vi "Principal.vi"() -> ()   [LabVIEW 2018]
panel:
  out "Turner Indicator":dbl(knob) scale=80.0..120.0 scale format="%#_50g"
  out "SHARP":bool
  out "TUNED":bool
  out "FLAT":bool
  in  "Choosing the string":i32(knob) scale=0.0..5.0
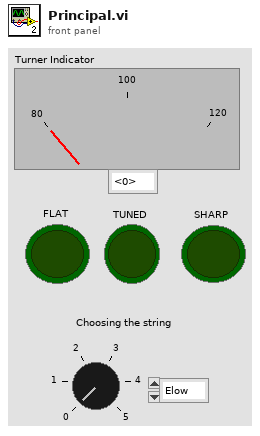
[diagram p1: front panel]
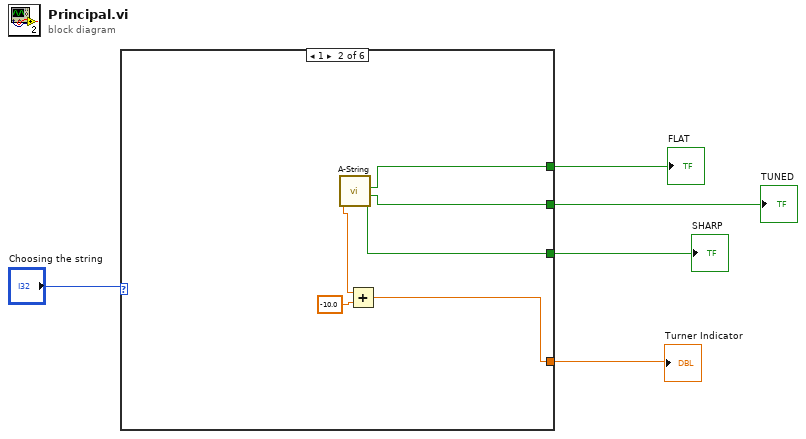
[diagram p0: block diagram]
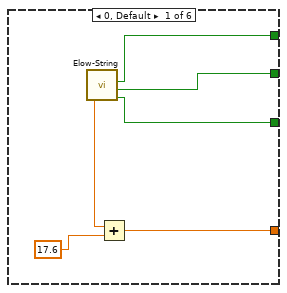
[diagram p2: hidden frame]
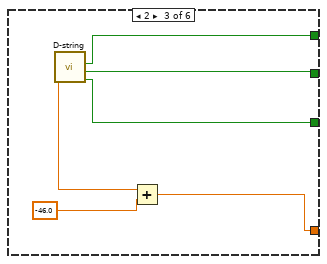
[diagram p3: hidden frame]
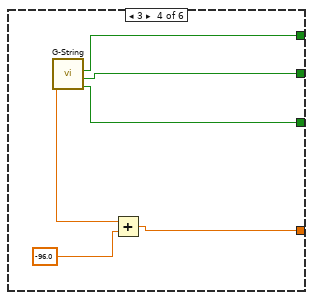
[diagram p4: hidden frame]
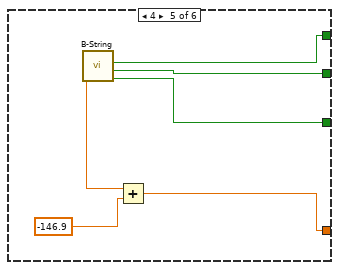
[diagram p5: hidden frame]
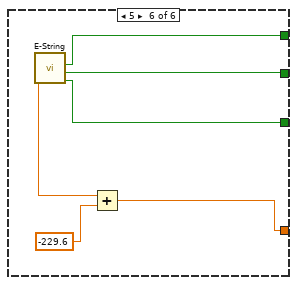
[diagram p6: hidden frame]
diagram:
  n1 = case shown="1" "Choosing the string" {
    tunnel: [w10 w16 w22 w26 w31 w38] -> w4
    tunnel: [w9 w15 w19 w29 w33 w41] -> w3
    tunnel: [w8 w14 w20 w28 w34 w40] -> w2
    tunnel: [w7 w13 w21 w27 w35 w39] -> w1
    frame 0, Default {
      n2 = call "Elow-String.vi"() -> ("SHARP"=w7:bool, "TUNED"=w8:bool, "FLAT"=w9:bool, "FREQ at maximum"=w6:dbl)  [unwired: 3 in, 1 out]
      n3 = Add(x=w6, y=17.6) -> (x+y=w10:dbl)
    }
    frame 1 {
      n4 = call "A-String.vi"() -> ("SHARP"=w13:bool, "TUNED"=w14:bool, "FLAT"=w15:bool, "FREQ at maximum"=w12:dbl)  [unwired: 6 in, 1 out]
      n5 = Add(x=w12, y=-10.0) -> (x+y=w16:dbl)
    }
    frame 2 {
      n6 = call "D-string.vi"() -> ("SHARP"=w21:bool, "TUNED"=w20:bool, "FLAT"=w19:bool, "FREQ at maximum"=w18:dbl)  [unwired: 7 in, 1 out]
      n7 = Add(x=w18, y=-46.0) -> (x+y=w22:dbl)
    }
    frame 3 {
      n8 = call "G-String.vi"() -> ("SHARP"=w27:bool, "TUNED"=w28:bool, "FLAT"=w29:bool, "FREQ at maximum"=w24:dbl)  [unwired: 5 in, 1 out]
      n9 = Add(x=w24, y=-96.0) -> (x+y=w26:dbl)
    }
    frame 4 {
      n10 = call "B-String.vi"() -> ("SHARP"=w35:bool, "TUNED"=w34:bool, "FLAT"=w33:bool, "FREQ at maximum"=w30:dbl)  [unwired: 5 in, 1 out]
      n11 = Add(x=w30, y=-146.9) -> (x+y=w31:dbl)
    }
    frame 5 {
      n12 = call "E-String.vi"() -> ("SHARP"=w39:bool, "TUNED"=w40:bool, "FLAT"=w41:bool, "FREQ at maximum"=w36:dbl)  [unwired: 6 in, 1 out]
      n13 = Add(x=w36, y=-229.6) -> (x+y=w38:dbl)
    }
  }
  "FLAT" <- w3
  "TUNED" <- w2
  "SHARP" <- w1
  "Turner Indicator" <- w4
